vi "Srednia FVG.vi"(6 "length (3)":i32=3, 8 "error in (no error)":errorcluster, 10 "temperatura in":dbl) -> (0 "error out":errorcluster, 2 "temperatura out":dbl, 3 "średnia out":dbl)   [LabVIEW 2013]
doc: "Liczy średnią z pomiarów\nStruktura pliku FVG"
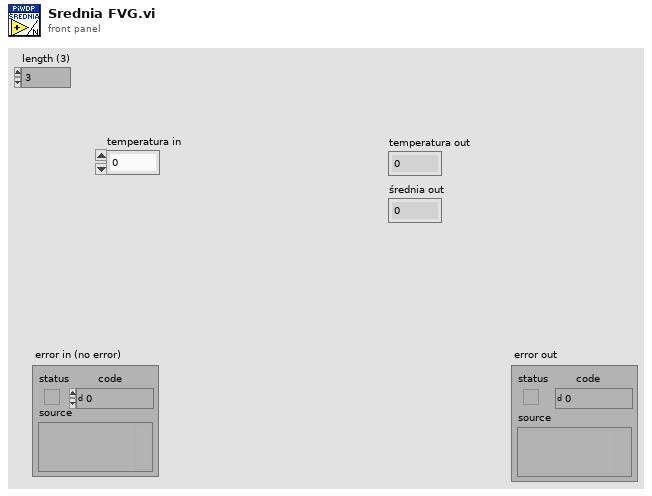
[diagram p1: front panel]
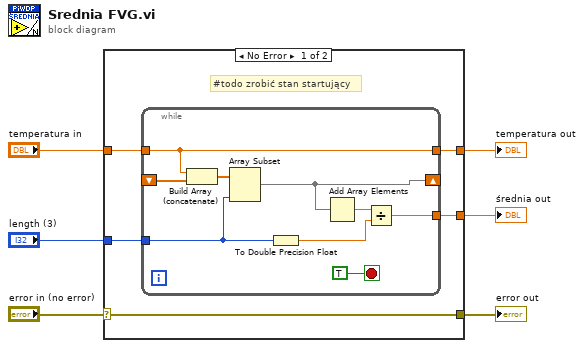
[diagram p0: block diagram]
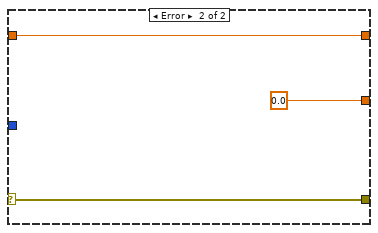
[diagram p2: hidden frame]
diagram:
  n1 = case shown="No Error" "error in (no error)" {
    selector: "error in (no error)" -> [w11 w23]
    tunnel: [w11 w23] -> w5
    tunnel: "temperatura in" -> [w10 w22]
    tunnel: "length (3)" -> [w9 _]
    tunnel: [w8 w22] -> w2
    tunnel: [w7 0.0] -> w1
    frame No Error {
      # "#todo zrobić stan startujący"
      n2 = while {
        tunnel: w10 -> [w17]
        tunnel: w9 -> [w14]
        shift-right: [w16] -> _
        shift-left: _ -> [w18]
        tunnel: [w17] -> w8
        tunnel: [w12] -> w7
        stop <- TRUE stop-if-true
        n3 = Build Array (concatenate)(w17, w18) -> (w19:dbl[])
        n4 = Array Subset(array=w19, length=w14) -> (w16:dbl[])  [unwired: 1 in]
        n5 = To Double Precision Float(number=w14) -> (double precision float=w13:dbl)
        n6 = Add Array Elements(numeric array=w16) -> (sum=w15:dbl)
        n7 = Divide(x=w15, y=w13) -> (x/y=w12:dbl)
      }
    }
    frame Error {
    }
  }
  "error out" <- w5
  "temperatura out" <- w2
  "średnia out" <- w1
